vi "SVM_matlab.vi"(7 "svm_parameter":T1={"svm_type"=0, "kernel_type"=3, "degree"=3, "gamma"=0.07, "coef0"=0.0, "cache_size"=100.0, "epsilon"=0.001, "C"=1.0, "nr_weight"=0, "weight_label"=[1, 12], "Weight (C(class i))"=[1.0, -1.0], "nu"=0.5, "p"=0.1, "Shrinking"=1, "probability"=1} {"p" format="%.4f"; "nu" format="%.4f"; "Weight (C(class i))" format="%.2f"; "C" format="%.2f"; "epsilon" format="%.4f"; "cache_size" format="%.2f"; "coef0" format="%.2f"; "gamma" format="%.5f"; "kernel_type" items=["Linear", "Poly", "RBF", "Sigmoid"]; "svm_type" items=["C-SVC", "Nu-SVC", "One-class SVM", "epsilon-SVR", "nu-SVR"]}, 8 "Target_total2 (from offline file)":path, 9 "ERP_all_icon (Online Data from offline file)":path, 10 "ERP_Parameters_of_NonTarget_prior":path, 11 "ERP_Parameters_of_Target_prior.txt":path) -> ()   [LabVIEW 2014]
uses:
  <vilib>/Utility/file.llb/Read From Spreadsheet File (DBL).vi
panel:
  out "selected_all":i16[](array[numeric])
  out "test predict":dbl[](array[numeric])=[-1.0, -1.0, -1.0, -1.0, -1.0, -1.0, -1.0, -1.0, -1.0, -1.0, -1.0, -1.0, -1.0, -1.0, -1.0, -1.0, -1.0, -1.0, -1.0, -1.0, -1.0, -1.0, -1.0, -1.0, 1.0, -1.0, 1.0, 1.0, -1.0, 1.0, -1.0, -1.0, -1.0, -1.0, -1.0, -1.0, 1.0, -1.0, 1.0, -1.0, 1.0, -1.0, -1.0, -1.0]
  out "Squared correlation\n coefficient":dbl
  out "Total":i32
  out "correct":i16
  out "Accuracy(%)":dbl
  in  "ModelFileName":string="C:\\\\WORK\\\\RBFModel"
  out "Length":i32=12
  # "Results"
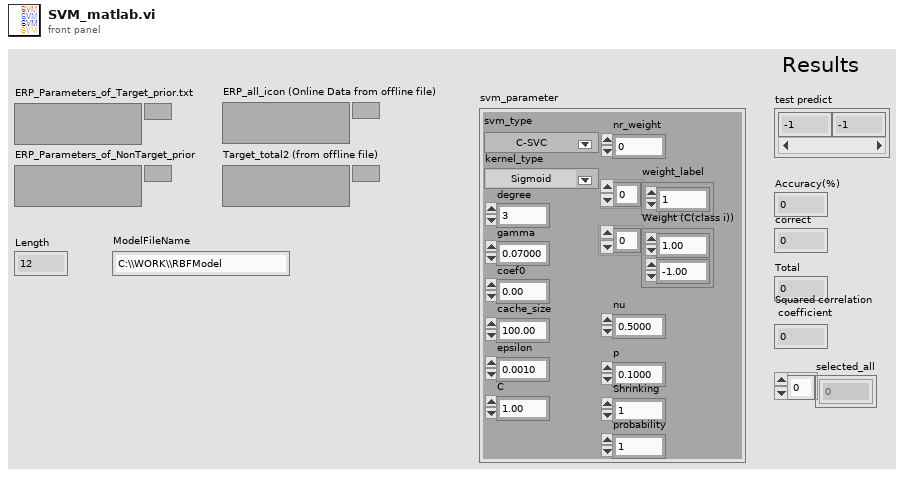
[diagram p1: front panel]
types:
  T1 = cluster{"svm_type":i16, "kernel_type":i16, "degree":i16, "gamma":dbl, "coef0":dbl, "cache_size":dbl, "epsilon":dbl, "C":dbl, "nr_weight":i16, "weight_label":i16[], "Weight (C(class i))":dbl[], "nu":dbl, "p":dbl, "Shrinking":i16, "probability":i16}
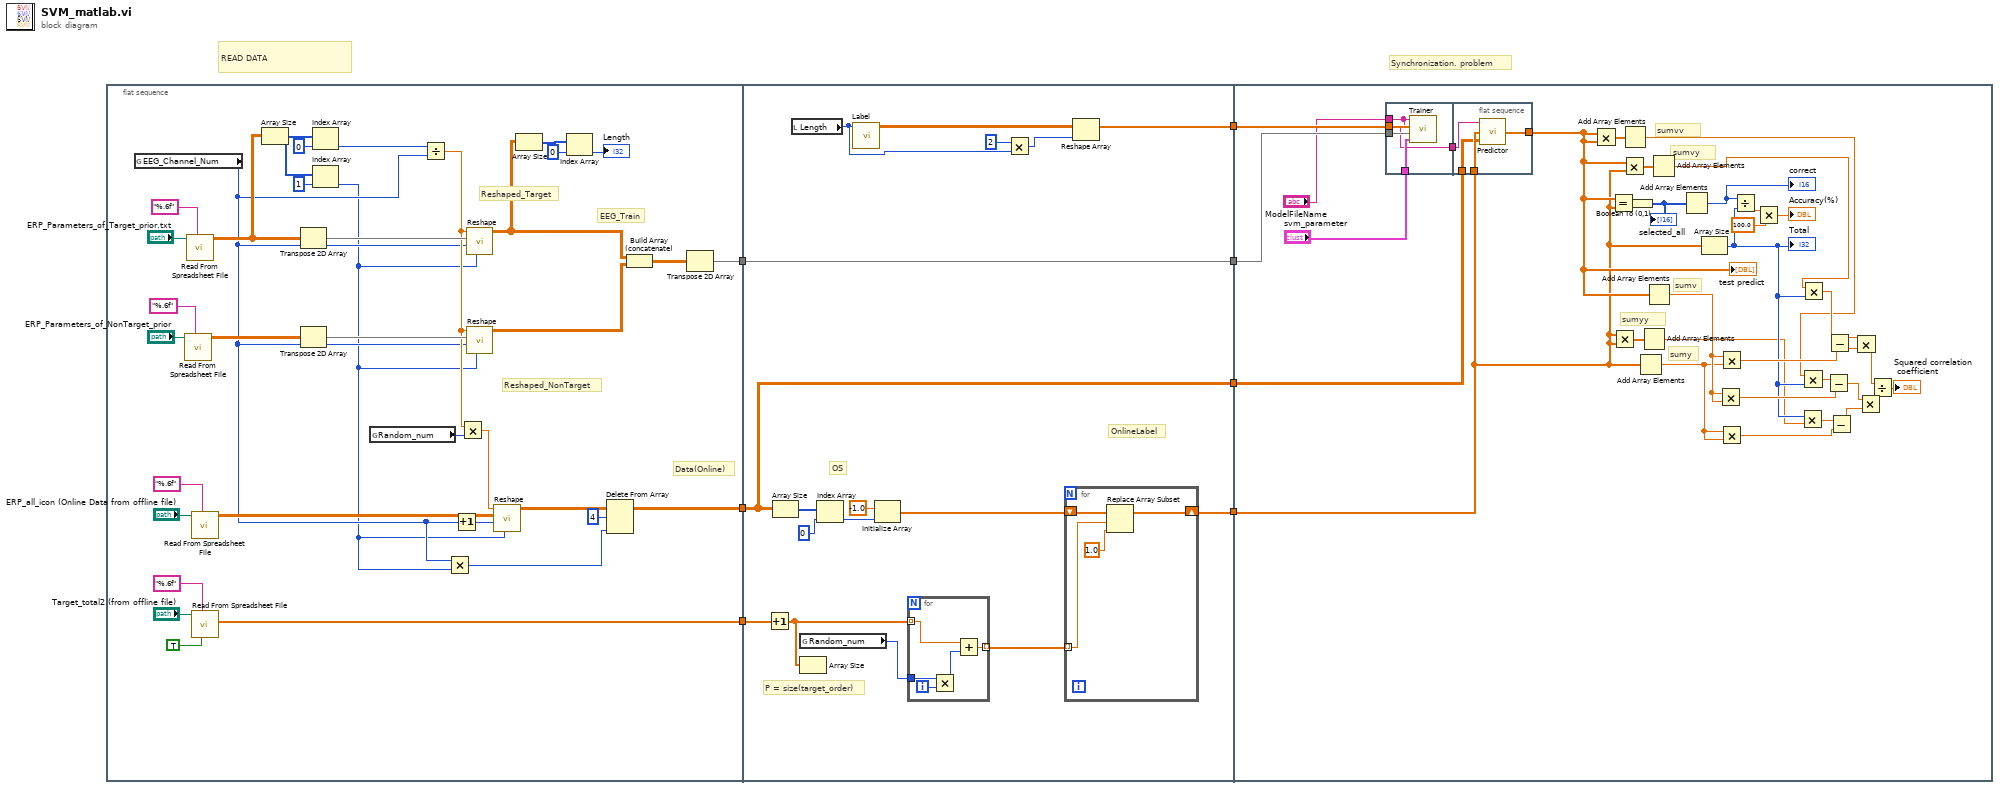
[diagram p0: block diagram]
diagram:
  # "Synchronization. problem"
  # "READ DATA"
  n1 = flat-sequence {
    tunnel: [w28] -> w7
    tunnel: [w15] -> w6
    tunnel: [w14] -> w5
    tunnel: w7 -> [w51]
    tunnel: w6 -> [w48]
    tunnel: w5 -> [w58]
    tunnel: [w51] -> w4
    tunnel: [w47] -> w3
    tunnel: [w49] -> w2
    tunnel: [w48] -> w1
    tunnel: w4 -> [w103]
    tunnel: w3 -> [w104]
    tunnel: w2 -> [w70]
    tunnel: w1 -> [w99]
    frame #0 {
      # "Data(Online)"
      # "EEG_Train"
      # "Reshaped_NonTarget"
      # "Reshaped_Target"
      n2 = global read "Control_Panel.vi" "EEG_Channel_Num"() -> (w17:i32)
      n3 = call-poly <vilib>:"Read From Spreadsheet File.vi"("format (%.3f)"="%.6f", "file path (dialog if empty)"="ERP_Parameters_of_NonTarget_prior") -> ("all rows"=w39:dbl[][])  [unwired: 5 in, 4 out]
      n4 = call-poly <vilib>:"Read From Spreadsheet File.vi"("format (%.3f)"="%.6f", "file path (dialog if empty)"="ERP_Parameters_of_Target_prior.txt") -> ("all rows"=w37:dbl[][])  [unwired: 5 in, 4 out]
      n5 = call-poly <vilib>:"Read From Spreadsheet File.vi"("format (%.3f)"="%.6f", "file path (dialog if empty)"="ERP_all_icon (Online Data from offline file)") -> ("all rows"=w22:dbl[][])  [unwired: 5 in, 4 out]
      n6 = call-poly <vilib>:"Read From Spreadsheet File.vi"("transpose (no:F)"=TRUE, "format (%.3f)"="%.6f", "file path (dialog if empty)"="Target_total2 (from offline file)") -> ("first row"=w14:dbl[])  [unwired: 4 in, 4 out]
      n7 = Array Size(array=w37) -> (size(s)=w35:i32[])
      n8 = Transpose 2D Array(2D array=w37) -> (transposed array=w31:dbl[][])
      n9 = Transpose 2D Array(2D array=w39) -> (transposed array=w30:dbl[][])
      n10 = Index Array(array=w35, index=0) -> (element=w34:i32)
      n11 = Index Array(array=w35, index=1) -> (element=w16:i32)
      n12 = global read "Control_Panel.vi" "Random_num"() -> (w21:i32)
      n13 = Divide(x=w34, y=w17) -> (x/y=w20:dbl)
      n14 = Multiply(x=w17, y=w16) -> (x*y=w11:i32)
      n15 = Increment(x=w17) -> (x+1=w18:i32)
      n16 = Multiply(x=w20, y=w21) -> (x*y=w19:dbl)
      n17 = call "Reshape.vi"("Numeric"=w16, "EEG_Channel_Num"=w17, "all rows"=w31, "Numeric 2"=w20) -> ("Array"=w10:dbl[][])  [unwired: 7 in]
      n18 = call "Reshape.vi"("Numeric"=w16, "EEG_Channel_Num"=w17, "all rows"=w30, "Numeric 2"=w20) -> ("Array"=w9:dbl[][])  [unwired: 7 in]
      n19 = call "Reshape.vi"("Numeric"=w16, "EEG_Channel_Num"=w18, "all rows"=w22, "Numeric 2"=w19) -> ("Array"=w12:dbl[][])  [unwired: 7 in]
      n20 = Array Size(array=w10) -> (size(s)=w32:i32[])
      n21 = Index Array(array=w32, index=0) -> (element=→"Length":i32)
      n22 = Delete From Array(array=w12, length=4, index (col)=w11) -> (array with subset deleted=w15:dbl[][])  [unwired: 1 in, 1 out]
      n23 = Build Array (concatenate)(w10, w9) -> (w8:dbl[][])
      n24 = Transpose 2D Array(2D array=w8) -> (transposed array=w28:dbl[][])
    }
    frame #1 {
      # "OnlineLabel"
      # "P = size(target_order)"
      # "OS"
      n25 = Increment(x=w58) -> (x+1=w57:dbl[])
      n26 = Array Size(array=w48) -> (size(s)=w60:i32[])
      n27 = local read "Length"() -> (w45:i32)
      n28 = global read "Control_Panel.vi" "Random_num"() -> (w56:i32)
      n29 = Array Size(array=w57) -> ()  [unwired: 1 out]
      n30 = Index Array(array=w60, index=0) -> (element=w55:i32)
      n31 = call "Label.vi"("Numeric"=w45) -> ("Array"=w50:dbl[][])  [unwired: 10 in]
      n32 = Initialize Array(-1.0 ("element"), w55) -> (w52:dbl[])
      n33 = for {
        tunnel: w57 -> [w66] mode=indexing
        tunnel: w56 -> [w68]
        tunnel: [w65] -> w53 mode=indexing
        i -> [w69]
        n34 = Multiply(x=w68, y=w69) -> (x*y=w67:i32)
        n35 = Add(x=w66, y=w67) -> (x+y=w65:dbl)
      }
      n36 = Multiply(x=2, y=w45) -> (x*y=w46:i32)
      n37 = for {
        tunnel: w53 -> [w63] mode=indexing
        shift-right: [w61] -> w49
        shift-left: w52 -> [w64]
        n38 = Replace Array Subset(array=w64, new element=1.0 ("new element/subarray"), index=w63) -> (w61:dbl[])
      }
      n39 = Reshape Array(w50, w46) -> (w47:dbl[])
    }
    frame #2 {
      # "sumyy"
      # "sumvy"
      # "sumvv"
      # "sumy"
      # "sumv"
      n40 = flat-sequence {
        tunnel: w104 -> [w108]
        tunnel: w103 -> [w107]
        tunnel: "ModelFileName" -> [w105]
        tunnel: "svm_parameter" -> [w106]
        tunnel: [w105] -> w100
        tunnel: w100 -> [w112]
        tunnel: w70 -> [w111]
        tunnel: w99 -> [w110]
        tunnel: [w109] -> w71
        frame #0 {
          n41 = call "Trainer.vi"("svm_parameter"=w106, "attributes"=w107, "Lables"=w108, "ModelFileName"=w105) -> ()
        }
        frame #1 {
          n42 = call "Predictor.vi"("attributes"=w110, "Lables"=w111, "ModelFileName"=w112) -> ("predictedlevel"=w109:dbl[])
        }
      }
      n43 = Multiply(x=w71, y=w71) -> (x*y=w79:dbl[])
      n44 = Equal?(x=w71, y=w70) -> (x = y?=w74:bool[])
      n45 = Multiply(x=w70, y=w70) -> (x*y=w78:dbl[])
      n46 = Multiply(x=w71, y=w70) -> (x*y=w80:dbl[])
      n47 = Add Array Elements(numeric array=w79) -> (sum=w76:dbl)
      n48 = Boolean To (0,1)(Boolean=w74) -> (0, 1=w75:i16[])
      "selected_all" <- w75
      n49 = Add Array Elements(numeric array=w70) -> (sum=w88:dbl)
      n50 = Add Array Elements(numeric array=w78) -> (sum=w73:dbl)
      n51 = Add Array Elements(numeric array=w71) -> (sum=w91:dbl)
      n52 = Add Array Elements(numeric array=w80) -> (sum=w77:dbl)
      n53 = Add Array Elements(numeric array=w75) -> (sum=w72:i16)
      "correct" <- w72
      n54 = Array Size(array=w70) -> (size(s)=w81:i32)
      "Total" <- w81
      n55 = Multiply(x=w91, y=w91) -> (x*y=w90:dbl)
      n56 = Multiply(x=w91, y=w88) -> (x*y=w94:dbl)
      n57 = Multiply(x=w88, y=w88) -> (x*y=w87:dbl)
      n58 = Divide(x=w72, y=w81) -> (x/y=w98:dbl)
      n59 = Multiply(x=w98, y=100.0) -> (x*y=→"Accuracy(%)":dbl)
      n60 = Multiply(x=w81, y=w73) -> (x*y=w89:dbl)
      n61 = Multiply(x=w76, y=w81) -> (x*y=w92:dbl)
      n62 = Multiply(x=w77, y=w81) -> (x*y=w95:dbl)
      n63 = Subtract(x=w92, y=w90) -> (x-y=w86:dbl)
      n64 = Subtract(x=w95, y=w94) -> (x-y=w93:dbl)
      n65 = Subtract(x=w89, y=w87) -> (x-y=w85:dbl)
      n66 = Multiply(x=w93, y=w93) -> (x*y=w84:dbl)
      n67 = Multiply(x=w86, y=w85) -> (x*y=w83:dbl)
      n68 = Divide(x=w84, y=w83) -> (x/y=→"Squared correlation\n coefficient":dbl)
      "test predict" <- w71
    }
  }
